vi "Rename Digital Pattern.vi"(6 "OldVal":string, 8 "error in (no error)":errorcluster, 9 "NewVal":string, 10 "Page Data in":T1 {"Node Ptr" format="%.0x"}, 11 "State Queue in":string[](array[string])) -> (0 "error out":errorcluster, 2 "Page Data out":T1 {"Node Ptr" format="%.0x"}, 3 "State Queue out":string[](array[string]))   [LabVIEW 2015, in "Engine Simulation Toolkit System Explorer.lvlib"]
uses:
  Engine Simulation Toolkit System Explorer.lvlib
  Digital Patterns Page Data.ctl
  <vilib>/NI Veristand/Custom Device API/Custom Device Item Ref.ctl
  Digital Pattern.ctl
  Digital Pattern Base.ctl
  Digital Pattern Remove Edge.ctl
  Digital Pattern Add Pulse.ctl
  <vilib>/NI Veristand/Custom Device API/Custom Device API.lvlib
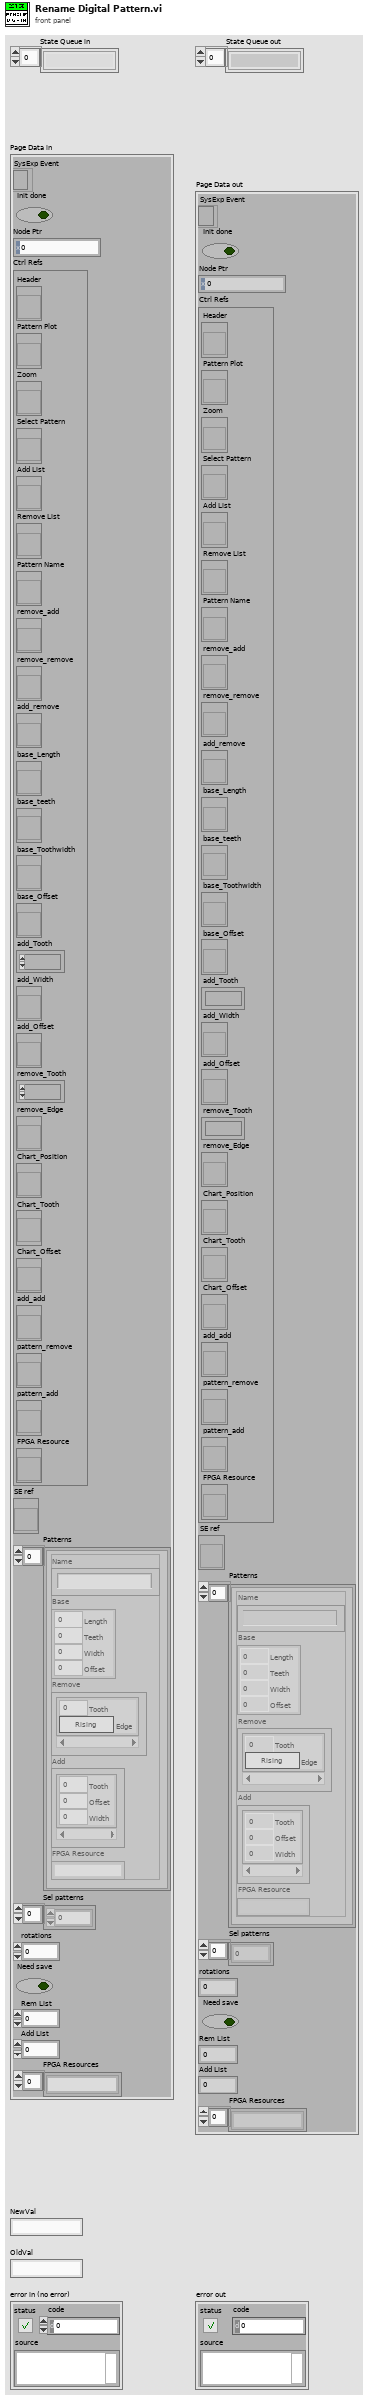
[diagram p1: front panel]
types:
  T1 = typedef "Engine Simulation Toolkit System Explorer.lvlib/Digital Patterns Page Data.ctl" = cluster{"SysExp Event":refnum<event-registration>, "Init done":bool, "Node Ptr":T2, "Ctrl Refs":cluster{"Header":refnum<vi>, "Pattern Plot":refnum<vi>, "Zoom":refnum<vi>, "Select Pattern":refnum<vi>, "Add List":refnum<vi>, "Remove List":refnum<vi>, "Pattern Name":refnum<vi>, "remove_add":refnum<vi>, "remove_remove":refnum<vi>, "add_remove":refnum<vi>, "base_Length":refnum<vi>, "base_teeth":refnum<vi>, "base_Toothwidth":refnum<vi>, "base_Offset":refnum<vi>, "add_Tooth":refnum<vi>, "add_Width":refnum<vi>, "add_Offset":refnum<vi>, "remove_Tooth":refnum<vi>, "remove_Edge":refnum<vi>, "Chart_Position":refnum<vi>, "Chart_Tooth":refnum<vi>, "Chart_Offset":refnum<vi>, "add_add":refnum<vi>, "pattern_remove":refnum<vi>, "pattern_add":refnum<vi>, "FPGA Resource":refnum<vi>}, "SE ref":refnum<vi>, "Patterns":T3[], "Sel patterns":i32[], "rotations":u16, "Need save":bool, "Rem List":i32, "Add List":i32, "FPGA Resources":string[]}
  T2 = typedef "Custom Device API.lvlib/Custom Device Item Ref.ctl" = u64
  T3 = typedef "Engine Simulation Toolkit System Explorer.lvlib/Digital Pattern.ctl" = cluster{"Name":string, "Base":T4, "Remove":T5[], "Add":T6[], "FPGA Resource":string}
  T4 = typedef "Engine Simulation Toolkit System Explorer.lvlib/Digital Pattern Base.ctl" = cluster{"Length":dbl, "Teeth":u16, "Width":dbl, "Offset":dbl}
  T5 = typedef "Engine Simulation Toolkit System Explorer.lvlib/Digital Pattern Remove Edge.ctl" = cluster{"Tooth":u16, "Edge":bool}
  T6 = typedef "Engine Simulation Toolkit System Explorer.lvlib/Digital Pattern Add Pulse.ctl" = cluster{"Tooth":u16, "Offset":dbl, "Width":dbl}
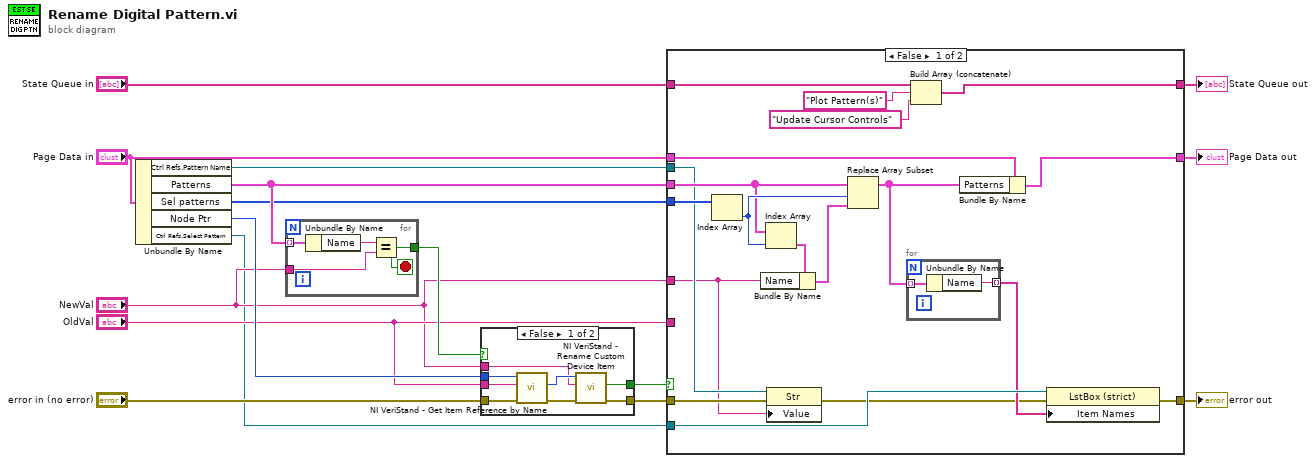
[diagram p0: block diagram]
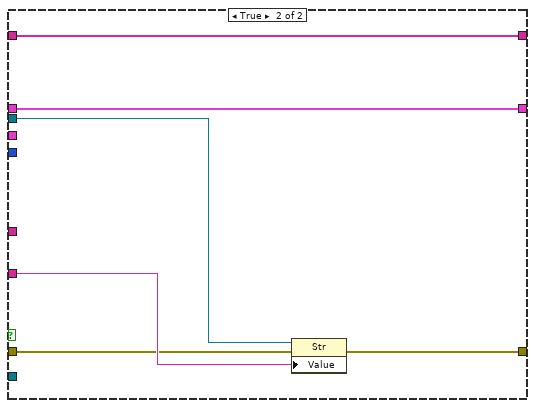
[diagram p3: hidden frame]
diagram:
  n1 = Unbundle By Name("Page Data in") -> ("Ctrl Refs.Pattern Name"=w9:refnum<vi>, "Patterns"=w15:T3[], "Sel patterns"=w11:i32[], "Node Ptr"=w7:T2, "Ctrl Refs.Select Pattern"=w1:refnum<vi>)
  n2 = for {
    tunnel: w15 -> [w20] mode=indexing
    tunnel: "NewVal" -> [w18]
    tunnel: [w17] -> w8
    stop <- w17 stop-if-true
    n3 = Unbundle By Name(w20) -> ("Name"=w19:string)
    n4 = Equal?(x=w19, y=w18) -> (x = y?=w17:bool)
  }
  n5 = case shown="False" w8 {
    selector: w8 -> [_ w29]
    tunnel: "error in (no error)" -> [w27 w30]
    tunnel: w7 -> [w26 _]
    tunnel: [w24 w30] -> w6
    tunnel: "OldVal" -> [w23 _]
    tunnel: "NewVal" -> [w22 _]
    tunnel: [w21 w29] -> w2
    frame False {
      n6 = call <vilib>:"NI VeriStand - Get Item Reference by Name.vi"("error in (no error)"=w27, "Item Name"=w23, "Parent Ref in"=w26) -> ("error out"=w25:errorcluster, "Item Ref"=w28:T2)  [unwired: 5 in, 2 out]
      n7 = call <vilib>:"NI VeriStand - Rename Custom Device Item.vi"("error in (no error)"=w25, "New Name"=w22, "Item Ref in"=w28) -> ("error out"=w24:errorcluster, "Request invalid?"=w21:bool)  [unwired: 6 in, 1 out]
    }
    frame True {
    }
  }
  n8 = case shown="False" w2 {
    tunnel: "State Queue in" -> [w49 w56]
    tunnel: w15 -> [w45 _]
    tunnel: w11 -> [w44 _]
    tunnel: "Page Data in" -> [w43 w55]
    tunnel: [w42 w55] -> w13
    tunnel: [w41 w56] -> w14
    tunnel: "OldVal" -> [_ w57]
    tunnel: "NewVal" -> [w31 _]
    tunnel: [w37 w52] -> w16
    tunnel: w6 -> [w34 w53]
    tunnel: w9 -> [w32 w54]
    tunnel: w1 -> [w36 _]
    frame False {
      n9 = Index Array(array=w44) -> (element=w46:i32)  [unwired: 1 in]
      n10 = Index Array(array=w45, index=w46) -> (element=w47:T3)
      n11 = Bundle By Name(cluster=w47, "Name"=w31) -> (w48:T3)
      n12 = property class="Str"(reference=w32, error in=w34, "Value"=w31) -> (error out=w33:errorcluster)  [unwired: 1 out]
      n13 = Replace Array Subset(array=w45, new element=w48, index=w46) -> (w38:T3[])
      n14 = for {
        tunnel: w38 -> [w51] mode=indexing
        tunnel: [w50] -> w35 mode=indexing
        n15 = Unbundle By Name(w51) -> ("Name"=w50:string)
      }
      n16 = Build Array (concatenate)(w49, "Plot Pattern(s)", "Update Cursor Controls") -> (w41:string[])
      n17 = Bundle By Name(cluster=w43, "Patterns"=w38) -> (w42:T1)
      n18 = property class="LstBox (strict)"(reference=w36, error in=w33, "Item Names"=w35) -> (error out=w37:errorcluster)  [unwired: 1 out]
    }
    frame True {
      n19 = property class="Str"(reference=w54, error in=w53, "Value"=w57) -> (error out=w52:errorcluster)  [unwired: 1 out]
    }
  }
  "error out" <- w16
  "State Queue out" <- w14
  "Page Data out" <- w13
